vi "New EnumeratedVariant.vi"(8 "error in (no error)":errorcluster, 9 "VEnum":variant, 10 "VData":variant, 11 "EnumeratedVariant in":refnum<class "EnumeratedVariant.lvclass">) -> (0 "error out":errorcluster, 3 "EnumeratedVariant out":refnum<class "EnumeratedVariant.lvclass">)   [LabVIEW 2020, in "EnumeratedVariant.lvclass"]
uses:
  EnumeratedVariant.lvclass
  EnumeratedVariant.lvclass/EnumeratedVariant.ctl
  Write VData.vi
  Write VEnum.vi
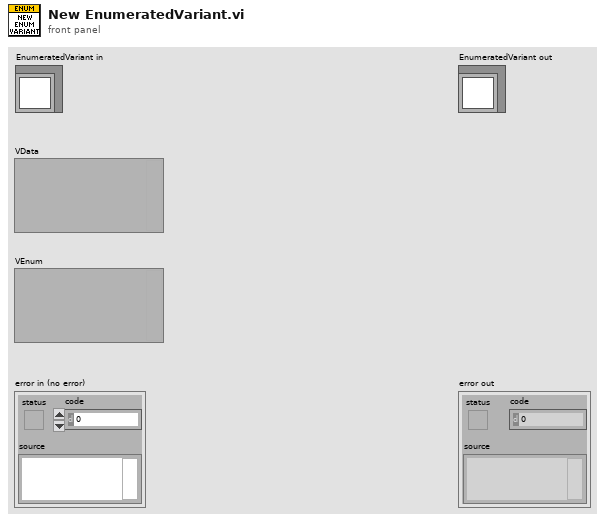
[diagram p1: front panel]
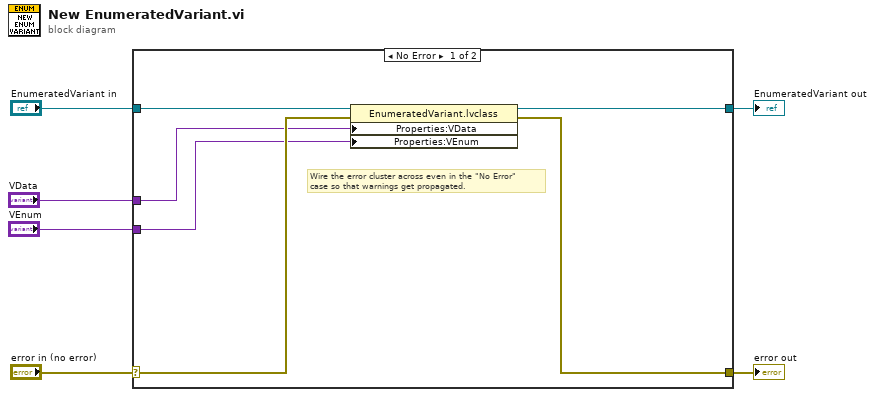
[diagram p0: block diagram]
diagram:
  n1 = case shown="No Error" "error in (no error)" {
    selector: "error in (no error)" -> [w10 w14]
    tunnel: [w9 w14] -> w5
    tunnel: [w11 w13] -> w3
    tunnel: "EnumeratedVariant in" -> [w12 w13]
    tunnel: "VData" -> [w8 _]
    tunnel: "VEnum" -> [w7 _]
    frame No Error {
      # "Wire the error cluster across even in the \"No Error\"\ncase so that warnings get propagated."
      n2 = property class="EnumeratedVariant.lvclass"(reference=w12, error in=w10, "Properties:VData"=w8, "Properties:VEnum"=w7) -> (reference out=w11:refnum<class "EnumeratedVariant.lvclass">, error out=w9:errorcluster)
    }
    frame Error {
    }
  }
  "error out" <- w5
  "EnumeratedVariant out" <- w3
